vi "TDC_getClockState.vi"(8 "Error In":errorcluster) -> (0 "Error Out":errorcluster, 1 "Uplink":bool, 2 "Locked":bool)   [LabVIEW 2011]
uses:
  tdcbase.dll
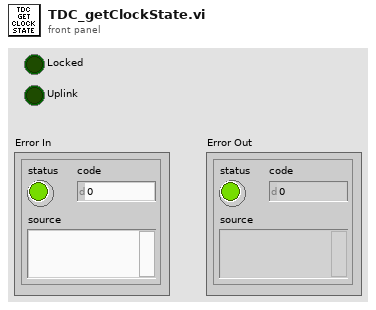
[diagram p1: front panel]
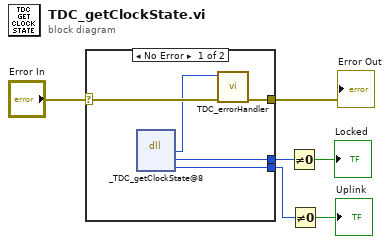
[diagram p0: block diagram]
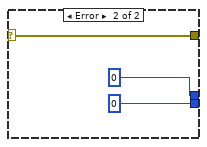
[diagram p2: hidden frame]
diagram:
  n1 = case shown="No Error" "Error In" {
    selector: "Error In" -> [w9 w14]
    tunnel: [w8 w14] -> w5
    tunnel: [w11 0] -> w4
    tunnel: [w10 0] -> w1
    frame No Error {
      n2 = dll-call lib="X:/tdcbase.dll" fn="_TDC_getClockState@8"() -> ("return type"=w7:i32, "locked"=w11:i32, "uplink"=w10:i32)  [unwired: 5 in, 2 out]
      n3 = call "TDC_errorHandler.vi"("Error In"=w9, "TDC Return Code"=w7) -> ("Error Out"=w8:errorcluster)  [unwired: 9 in]
    }
    frame Error {
    }
  }
  "Error Out" <- w5
  n4 = Not Equal To 0?(x=w4) -> (x != 0?=→"Locked":bool)
  n5 = Not Equal To 0?(x=w1) -> (x != 0?=→"Uplink":bool)
